vi "Fail condition test.vi"() -> ()   [LabVIEW 2013]
panel:
  in  "대기 시간(ms)":u32
  in  "pass/fail":bool[](array[boolean])
  in  "정지":bool
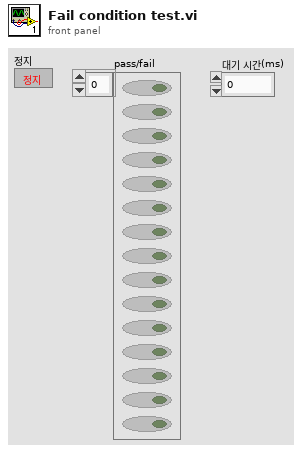
[diagram p1: front panel]
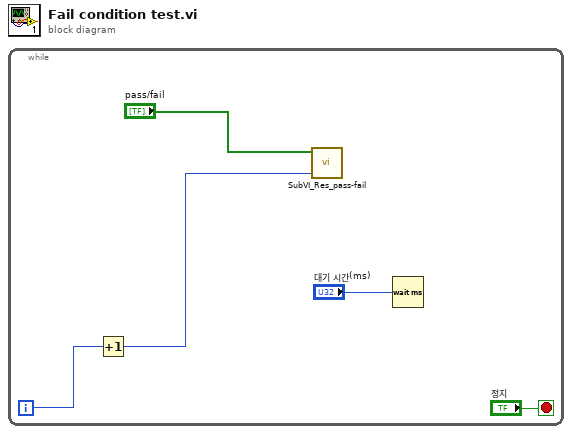
[diagram p0: block diagram]
diagram:
  n1 = while {
    i -> [w3]
    stop <- "정지" stop-if-true
    n2 = Increment(x=w3) -> (x+1=w2:i32)
    n3 = call "SubVI_Res_pass-fail.vi"("Current Cycle"=w2, "pass/fail"="pass/fail") -> ()  [unwired: 8 in, 2 out]
    n4 = Wait (ms)(milliseconds to wait="대기 시간(ms)") -> ()  [unwired: 1 out]
  }
